vi "drawField.vi"(0 "Vision in":refnum<class "Vision.lvclass">, 1 "AutoScale":bool=TRUE, 5 "Field State Input":T12 {"Detection Frame Out"."robots_blue"."height" format="%+4.3f"; "Detection Frame Out"."robots_blue"."pixel_y" format="%+4.3f"; "Detection Frame Out"."robots_blue"."pixel_x" format="%+4.3f"; "Detection Frame Out"."robots_blue"."orientation" format="%+4.3f"; "Detection Frame Out"."robots_blue"."y" format="%+4.3f"; "Detection Frame Out"."robots_blue"."confidence" format="%4.3f"; "Detection Frame Out"."robots_blue"."x" format="%+4.3f"; "Detection Frame Out"."robots_yellow"."height" format="%+4.3f"; "Detection Frame Out"."robots_yellow"."pixel_y" format="%+4.3f"; "Detection Frame Out"."robots_yellow"."pixel_x" format="%+4.3f"; "Detection Frame Out"."robots_yellow"."orientation" format="%+4.3f"; "Detection Frame Out"."robots_yellow"."y" format="%+4.3f"; "Detection Frame Out"."robots_yellow"."confidence" format="%4.3f"; "Detection Frame Out"."robots_yellow"."x" format="%+4.3f"}, 7 "AI Parameters":T17={"GotoKick"={"Dist do cone a frente"=0.0, "attacker farback"=1300.0, "Perto"=300.0, "min dist to kick"=140.0, "kick eps"=0.15, "Time to transition"=0.3}, "Attacker"={"CC chute"=0.7, "CC passe"=0.65, "Kick Force"=85.0, "ball-robot Kick"=300.0, "ball-robot Pass"=350.0, "drible\nAttk"=FALSE}, "Defender"={"D max"=1500.0, "Vel p/ robô av"=0.2, "Kick Force"=100.0, "D atk-def"=400.0, "D farback"=300.0, "drible\ndef"=FALSE, "drible\ngoalie"=FALSE}, "Timeout"={"Field/v in x"=6.0, "Dist Robots"=300, "Dist up in y"=300}, "Pose Striker"={"dist"=650.0, "Numeric"=-4.0, "dist 2"=650.0, "drible\nstriker"=TRUE}, "Dist Stop"=700.0, "D ball out"=200, "D central gap "=125.0, "T pass"=5.0, "Force ++"=5.0, "range kick"=60.0, "Chute alto"=TRUE, "Marcador novo"=TRUE, "drible"=FALSE, "D drible"=500.0, "Versão Striker"=enum."Auto", "Defesa"=enum."ManMark", "Marcador"=enum."Marcar o mais perigoso", "Receptor passe"=enum."Auto", "Área"=enum."Circular", "Decisão\nsimples?"=FALSE} {"D drible" format="%#_13g"; "D central gap" format="%#_13g"; "Dist Stop" format="%#_13g"; "Pose Striker"."Numeric" format="%#_13g"; "Defender"."Kick Force" format="%#_13g"; "Defender"."Vel p/ robô av" format="%#_13g"; "Attacker"."ball-robot Kick" format="%#_13g"; "Attacker"."Kick Force" format="%#_13g"; "Attacker"."CC passe" format="%#_13g"; "Attacker"."CC chute" format="%#_13g"; "GotoKick"."min dist to kick" format="%#_13g"; "GotoKick"."Perto" format="%#_13g"; "GotoKick"."attacker farback" format="%#_13g"; "GotoKick"."Dist do cone a frente" format="%#_13g"}, 9 "AI State":T1={"our_robots"=[], "enemy_robots"=[], "balls"=[], "geometry"={"line_width"=0, "field_length"=0, "field_width"=0, "boundary_width"=0, "referee_width"=0, "goal_width"=0, "goal_depth"=0, "goal_wall_width"=0, "center_circle_radius"=0, "defense_radius"=0, "defense_stretch"=0, "free_kick_from_defense_dist"=0, "penalty_spot_from_field_line_dist"=0, "penalty_line_from_spot_dist"=0}, "IA Judge"={"stage"="", "command"="", "our_goalie_id"=0.0, "enemy_goalie_id"=0.0, "command enum"=enum."Halt", "Time"=enum."Azul"}, "Received Timestamp"=timestamp(0 s since 1904-01-01), "Events"={"Touch"=FALSE, "Ball out"=FALSE, "id touch"=0.0, "Ball out of \nVision"=FALSE, "Ball inside \nGoalie area"=FALSE, "Robot not responding"=FALSE, "Robots responding status"=[1.0, 1.0, 1.0, 1.0, 1.0, 1.0], "Enemy Ball \nPossession"=FALSE, "Pass State"=FALSE, "id end of pass"=0.0, "Kick"=FALSE, "Id ini Possession"=0.0, "Ball Possesion"=FALSE, "Id Possesion"=0.0, "Direct Kick"=FALSE, "2nd Strk Ativo"=FALSE}}, 11 "error in (no error)":errorcluster, 12 "Scale mm/pixel":dbl=1.0 format="%#_13g", 13 "Draw Targets?":T18, 14 "Zoom":dbl) -> (3 "AutoScale Out":bool=TRUE, 4 "Vision out":refnum<class "Vision.lvclass">, 6 "2D Picture":picture, 10 "Scale Out":dbl, 15 "error out":errorcluster)   [LabVIEW 2018, in "Vision.lvclass"]
uses:
  Vision.lvclass
  git/SSLView/DrawTargets.ctl
  git/SSLView/Intel/AI Parameters.ctl
  Old vision/Controls/SSL Field State.ctl
  Old vision/Controls/SSL Detection Frame.ctl
  Old vision/Controls/SSL Detection Robot.ctl
  <vilib>/Analysis/Matrix/Datatypes/RealMatrix.ctl
  Old vision/Controls/SSL Detection Ball.ctl
  Old vision/Controls/AI Input.ctl
  Old vision/Controls/AI Robot.ctl
  Old vision/Controls/Functions Enum.ctl
  Old vision/Controls/AttackerStates.ctl
  Old vision/Controls/PathDests.ctl
  Old vision/Controls/PathDest.ctl
  Old vision/Controls/AI Ball.ctl
  Old vision/Controls/Field Size.ctl
  Old vision/Controls/AI Judge.ctl
  Old vision/Controls/Command Enum.ctl
  Old vision/Controls/Events.ctl
  <vilib>/Utility/miscctls.llb/LVBoundsTypeDef.ctl
  <vilib>/Analysis/Matrix/NI_Matrix.lvlib
panel:
  in  "Side":enum16{"Esquerdo", "Direito"}(ring) caption="Enum"
  in  "Defense stretch":i32=500
  in  "Defense width":i32=1000
  in  "Draw Number":bool=TRUE
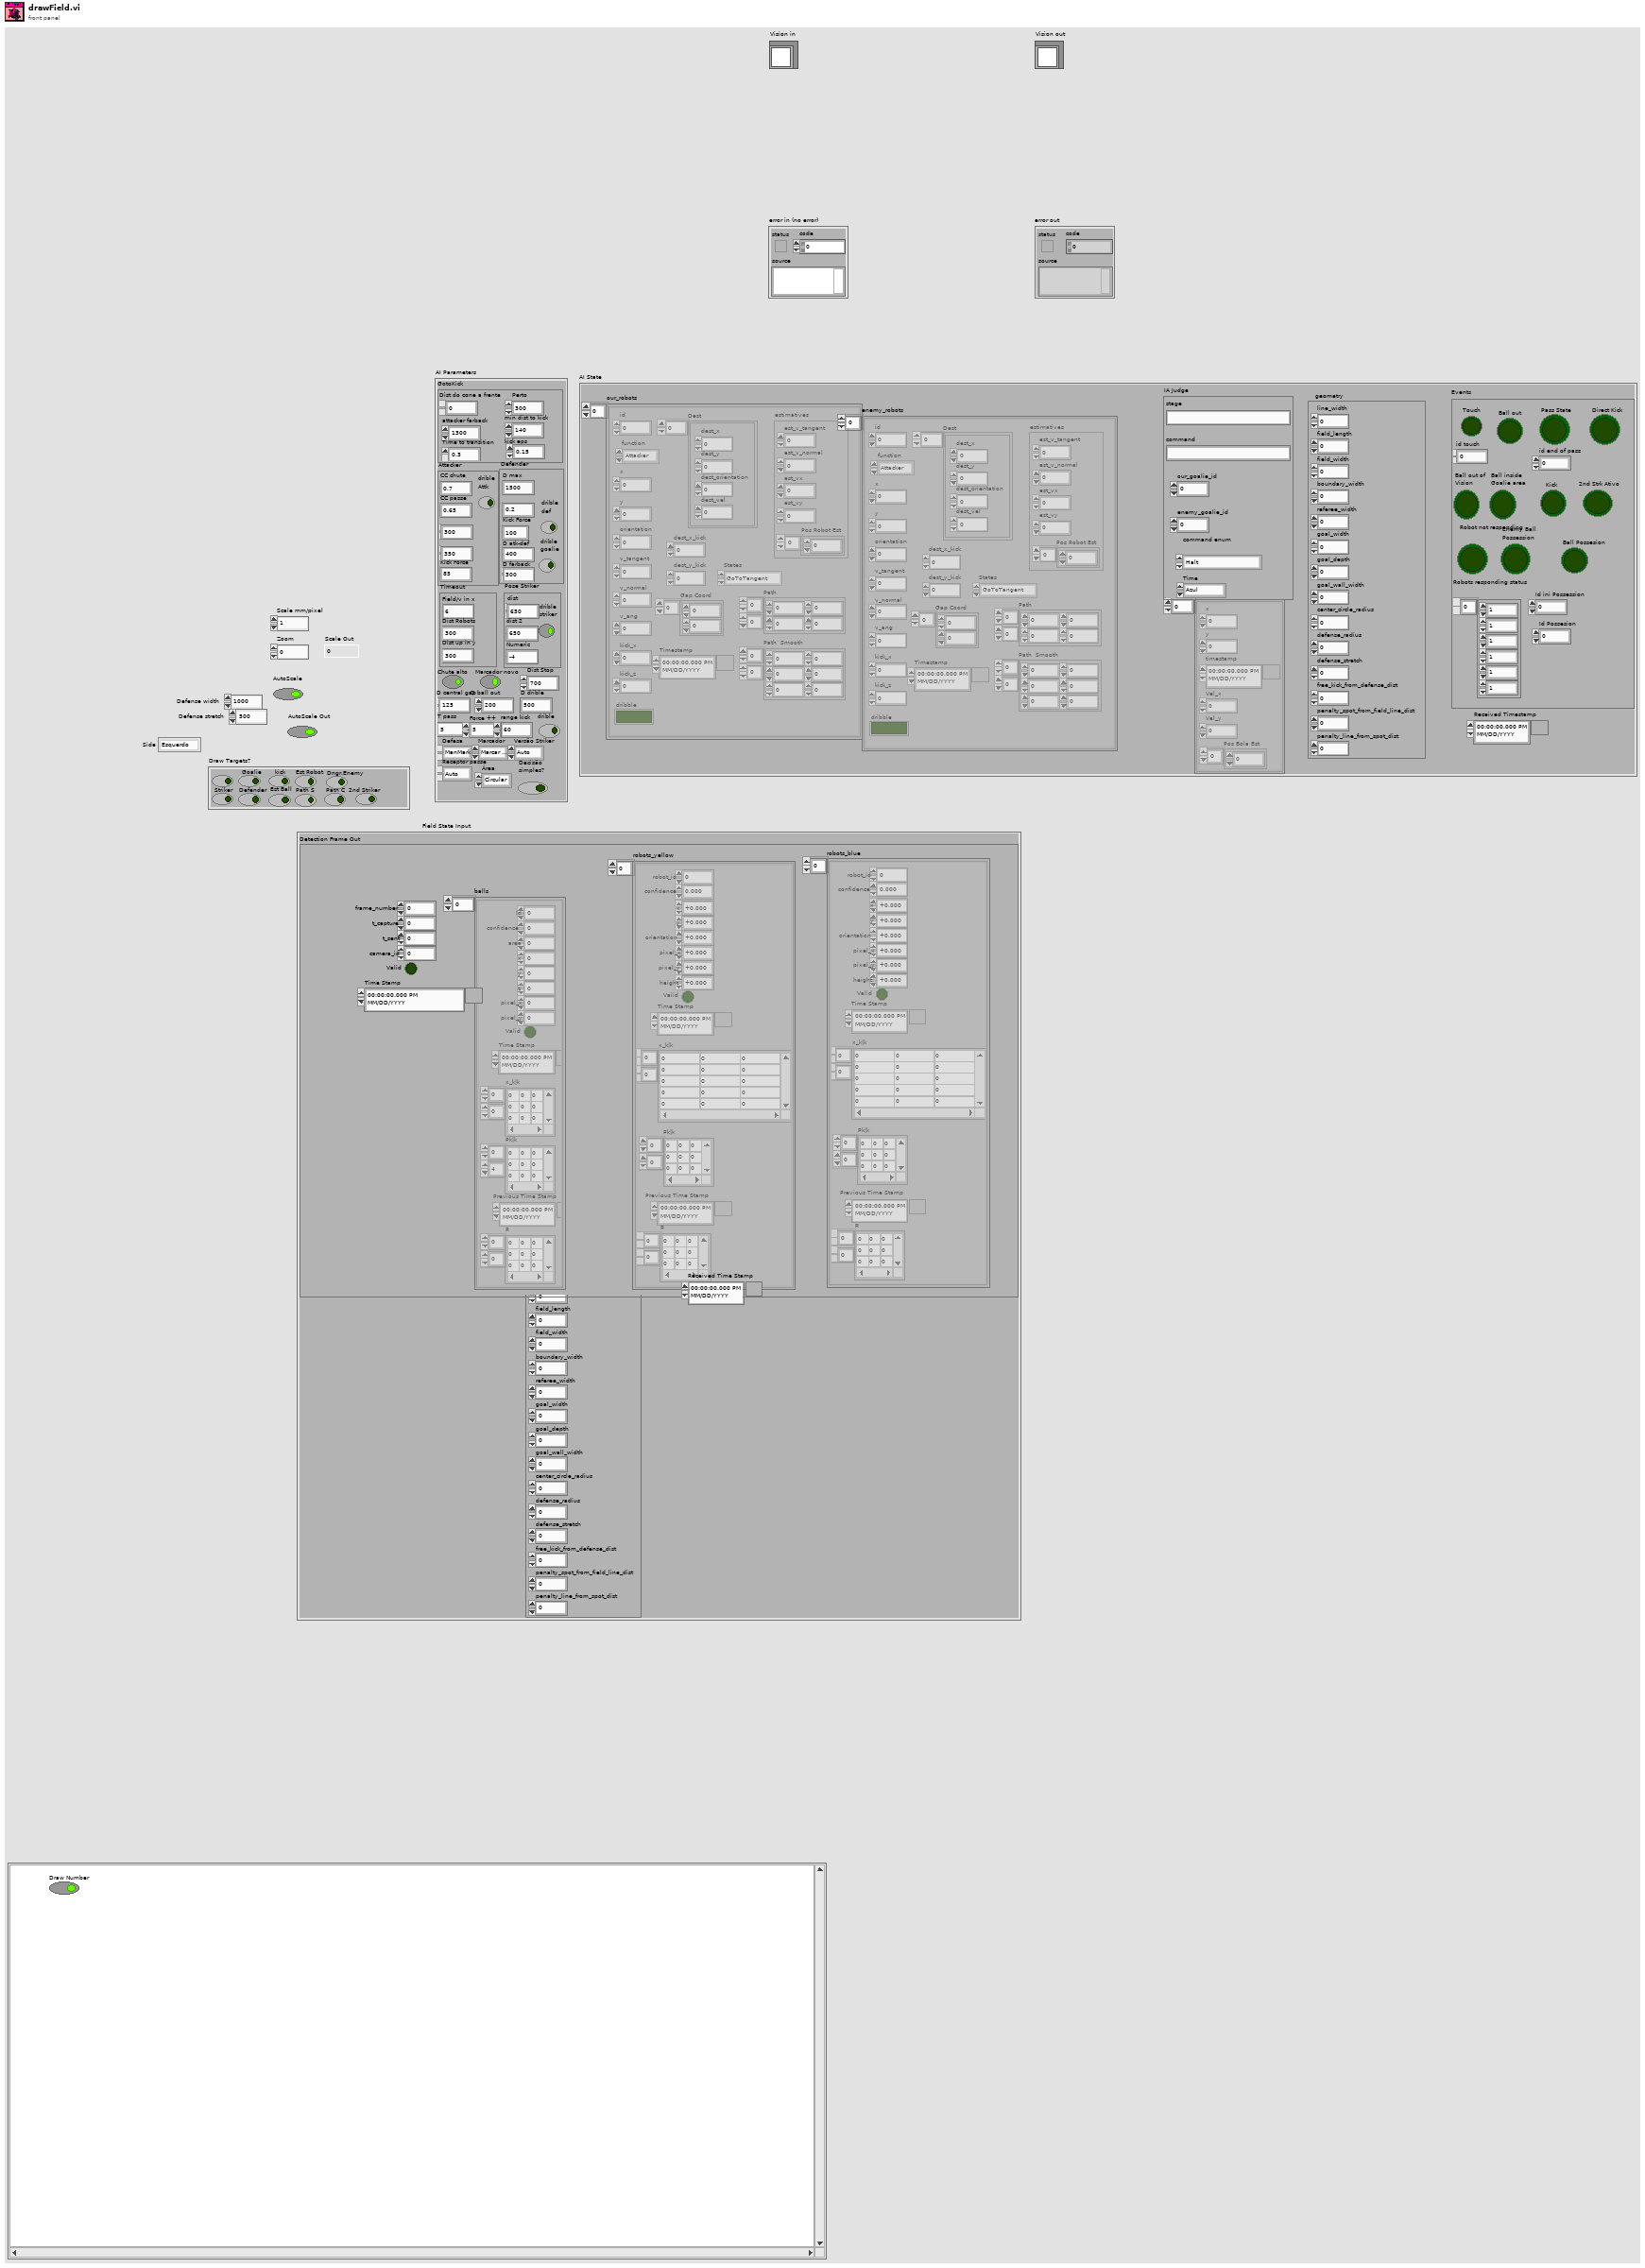
[diagram p1: front panel]
types:
  T1 = typedef "AI Input.ctl" = cluster{"our_robots":T2[], "enemy_robots":T2[], "balls":T7[], "geometry":T8, "IA Judge":T9, "Received Timestamp":timestamp, "Events":T11}
  T2 = typedef "AI Robot.ctl" = cluster{"id":u32, "function":T3, "x":dbl, "y":dbl, "orientation":dbl, "v_tangent":dbl, "v_normal":dbl, "v_ang":dbl, "kick_x":dbl, "kick_z":dbl, "dribble":bool, "Timestamp":timestamp, "estimatives":cluster{"est_v_tangent":dbl, "est_v_normal":dbl, "est_vx":dbl, "est_vy":dbl, "Pos Robot Est":dbl[]}, "dest_x_kick":dbl, "dest_y_kick":dbl, "Gap Coord":dbl[], "States":T4, "Path ":dbl[][], "Path  Smooth":dbl[][], "Dest":T5}
  T3 = typedef "Functions Enum.ctl" = enum16{"2nd Striker", "Attacker", "Goalie", "Defender", "Striker", "Goto 0", "Dummy", "Kicker", "ZigZag 0", "ZigZag 1", "ZigZag 2", "ZigZag 3", "ZigZag 4", "ZigZag 5", "ZigZag 6", "ZigZag 7", "ZigZag 8", ""}
  T4 = typedef "AttackerStates.ctl" = enum16{"Pass", "GoToTangent", "BallGetting", "GoToKick", ""}
  T5 = typedef "PathDests.ctl" = T6[]
  T6 = typedef "PathDest.ctl" = cluster{"dest_x":dbl, "dest_y":dbl, "dest_orientation":dbl, "dest_vel":dbl}
  T7 = typedef "AI Ball.ctl" = cluster{"x":dbl, "y":dbl, "timestamp":timestamp, "Vel_x":dbl, "Vel_y":dbl, "Pos Bola Est":dbl[]}
  T8 = typedef "Field Size.ctl" = cluster{"line_width":u32, "field_length":u32, "field_width":u32, "boundary_width":u32, "referee_width":u32, "goal_width":u32, "goal_depth":u32, "goal_wall_width":u32, "center_circle_radius":u32, "defense_radius":u32, "defense_stretch":u32, "free_kick_from_defense_dist":u32, "penalty_spot_from_field_line_dist":u32, "penalty_line_from_spot_dist":u32}
  T9 = typedef "AI Judge.ctl" = cluster{"stage":string, "command":string, "our_goalie_id":dbl, "enemy_goalie_id":dbl, "command enum":T10, "Time":enum16{"Azul", "Amarelo"}}
  T10 = typedef "Command Enum.ctl" = enum16{"Halt", "Stop", "Force Start", "PKA Normal Start", "Prepare Kickoff Ally", "PKE Normal Start", "Prepare Kickoff Enemy", "Prepare Penalty Ally", "PPA Normal Start", "Prepare Penalty Enemy", "PPE Normal Start", "Direct Free Enemy", "Direct Free Ally", "Indirect Free Enemy", "Indirect Free Ally", "Timeout Enemy", "Timeout Ally", "Goal Enemy", "Goal Ally", "Ball Placement Enemy", "Ball Placement Ally", "Normal Half Time", "Extra Time Break", "Extra Half Time", "None", "Post Game"}
  T11 = typedef "Events.ctl" = cluster{"Touch":bool, "Ball out":bool, "id touch":dbl, "Ball out of \nVision":bool, "Ball inside \nGoalie area":bool, "Robot not responding":bool, "Robots responding status":dbl[], "Enemy Ball \nPossession":bool, "Pass State":bool, "id end of pass":dbl, "Kick":bool, "Id ini Possession":dbl, "Ball Possesion":bool, "Id Possesion":dbl, "Direct Kick":bool, "2nd Strk Ativo":bool}
  T12 = typedef "SSL Field State.ctl" = cluster{"Detection Frame Out":T13, "Field Size Out":cluster{"line_width":u32, "field_length":u32, "field_width":u32, "boundary_width":u32, "referee_width":u32, "goal_width":u32, "goal_depth":u32, "goal_wall_width":u32, "center_circle_radius":u32, "defense_radius":u32, "defense_stretch":u32, "free_kick_from_defense_dist":u32, "penalty_spot_from_field_line_dist":u32, "penalty_line_from_spot_dist":u32}, "Received Time Stamp":timestamp}
  T13 = typedef "SSL Detection Frame.ctl" = cluster{"frame_number":u32, "t_capture":dbl, "t_sent":dbl, "camera_id":u32, "robots_yellow":T14[], "robots_blue":T14[], "balls":T16[], "Valid":bool, "Time Stamp":timestamp}
  T14 = typedef "SSL Detection Robot.ctl" = cluster{"x":sgl, "robot_id":u32, "confidence":sgl, "y":sgl, "orientation":sgl, "pixel_x":sgl, "pixel_y":sgl, "height":sgl, "Valid":bool, "Time Stamp":timestamp, "x_k|k":T15, "Pk|k":T15, "Previous Time Stamp":timestamp, "R":T15}
  T15 = typedef "NI_Matrix.lvlib/RealMatrix.ctl" = dbl[][]
  T16 = typedef "SSL Detection Ball.ctl" = cluster{"x":sgl, "area":u32, "confidence":sgl, "y":sgl, "z":sgl, "pixel_x":sgl, "pixel_y":sgl, "Valid":bool, "Time Stamp":timestamp, "x_k|k":T15, "Pk|k":T15, "Id":u32, "Previous Time Stamp":timestamp, "R":T15}
  T17 = typedef "AI Parameters.ctl" = cluster{"GotoKick":cluster{"Dist do cone a frente":dbl, "attacker farback":dbl, "Perto":dbl, "min dist to kick":dbl, "kick eps":dbl, "Time to transition":dbl}, "Attacker":cluster{"CC chute":dbl, "CC passe":dbl, "Kick Force":dbl, "ball-robot Kick":dbl, "ball-robot Pass":dbl, "drible\nAttk":bool}, "Defender":cluster{"D max":dbl, "Vel p/ robô av":dbl, "Kick Force":dbl, "D atk-def":dbl, "D farback":dbl, "drible\ndef":bool, "drible\ngoalie":bool}, "Timeout":cluster{"Field/v in x":dbl, "Dist Robots":u32, "Dist up in y":u32}, "Pose Striker":cluster{"dist":dbl, "Numeric":dbl, "dist 2":dbl, "drible\nstriker":bool}, "Dist Stop":dbl, "D ball out":i32, "D central gap ":dbl, "T pass":dbl, "Force ++":dbl, "range kick":dbl, "Chute alto":bool, "Marcador novo":bool, "drible":bool, "D drible":dbl, "Versão Striker":enum16{"Auto", "3", "2", "1"}, "Defesa":enum16{"ManMark", "Barreira"}, "Marcador":enum16{"Marcar Segundo mais perigoso", "Marcar o mais perigoso"}, "Receptor passe":enum16{"Auto", "2nd Striker", "Striker"}, "Área":enum16{"Quadrada", "Circular"}, "Decisão\nsimples?":bool}
  T18 = typedef "DrawTargets.ctl" = cluster{"Attacker":bool, "Striker":bool, "Goalie":bool, "Defender":bool, "kick":bool, "Est Ball":bool, "Est Robot":bool, "Path S":bool, "Path C":bool, "Dngr.Enemy":bool, "2nd Striker":bool}
  T19 = typedef "LVBoundsTypeDef.ctl" = cluster{"Width":u32, "Height":u32}
  T20 = cluster{"line_width":u32, "field_length":u32, "field_width":u32, "boundary_width":u32, "referee_width":u32, "goal_width":u32, "goal_depth":u32, "goal_wall_width":u32, "center_circle_radius":u32, "defense_radius":u32, "defense_stretch":u32, "free_kick_from_defense_dist":u32, "penalty_spot_from_field_line_dist":u32, "penalty_line_from_spot_dist":u32}
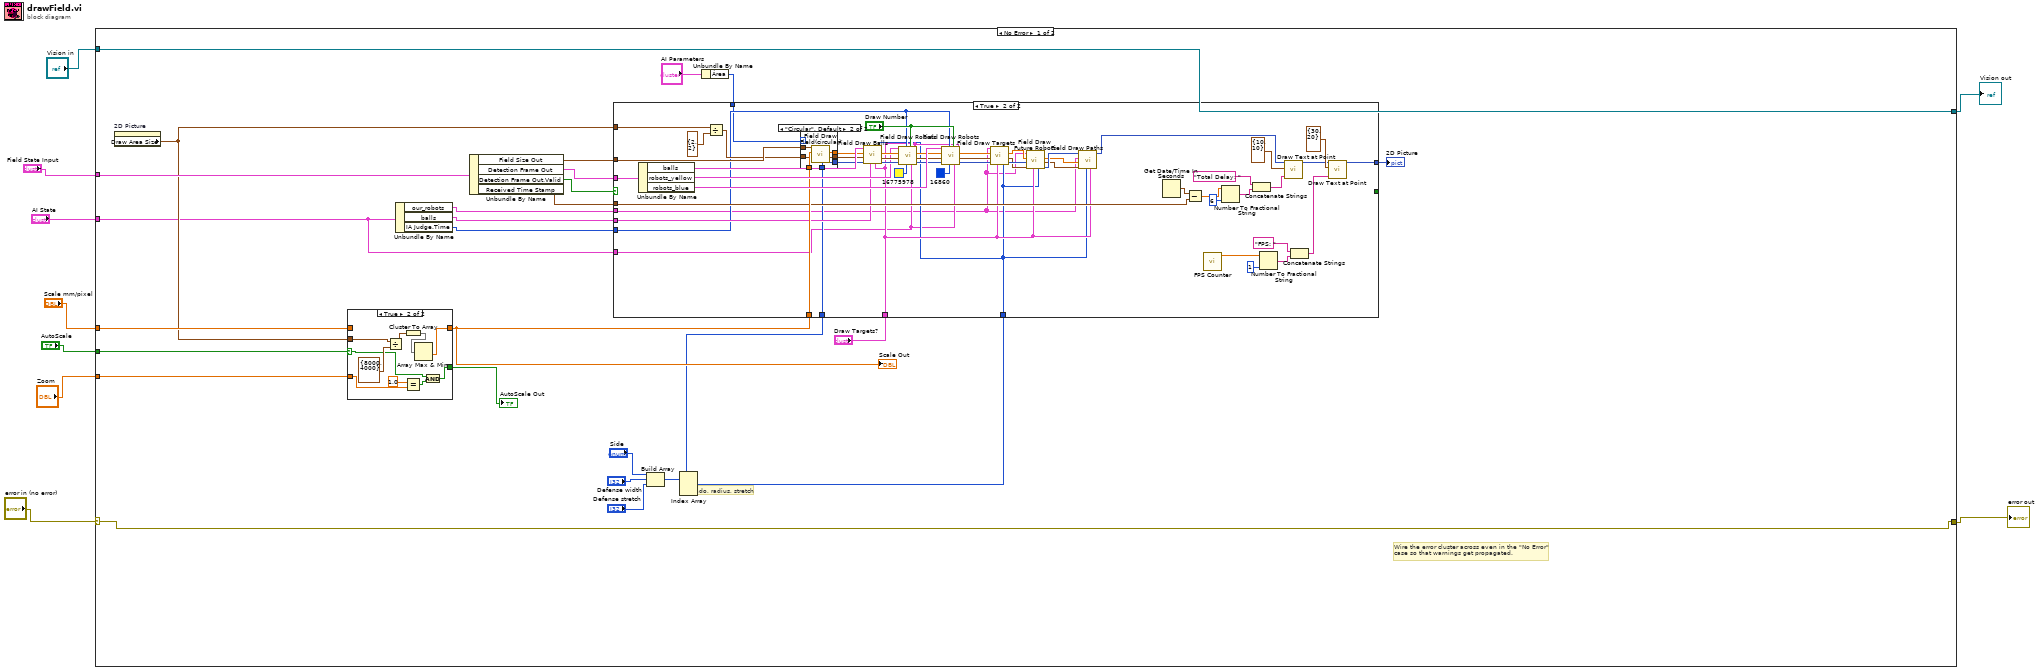
[diagram p0: block diagram]
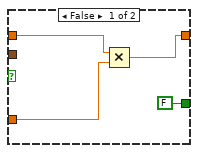
[diagram p2: hidden frame]
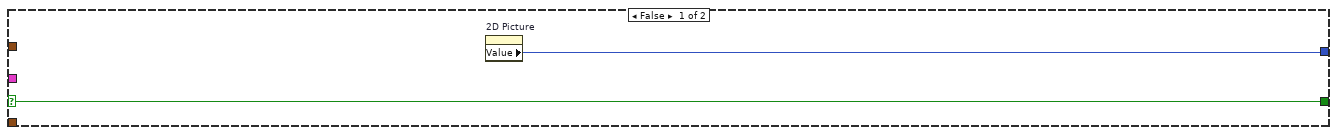
[diagram p3: hidden frame]
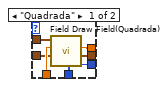
[diagram p4: hidden frame]
diagram:
  n1 = case shown="No Error" "error in (no error)" {
    selector: "error in (no error)" -> [w34 w122]
    tunnel: [w34 w122] -> w8
    tunnel: [w35 w121] -> w6
    tunnel: "Vision in" -> [w35 w121]
    tunnel: "Scale mm/pixel" -> [w24 _]
    tunnel: "AutoScale" -> [w23 _]
    tunnel: "Zoom" -> [w22 _]
    tunnel: "Field State Input" -> [w20 _]
    tunnel: "AI State" -> [w15 _]
    frame No Error {
      # "lado, radius, stretch"
      # "Wire the error cluster across even in the \"No Error\"\ncase so that warnings get propagated."
      n2 = property on="2D Picture" class="Pict"() -> ("Draw Area Size"=w16:T19)  [unwired: 2 in, 2 out]
      n3 = case shown="True" w23 {
        selector: w23 -> [_ w41]
        tunnel: w24 -> [w39 _]
        tunnel: [w38 w45] -> w14
        tunnel: w16 -> [_ w49]
        tunnel: w22 -> [w37 w44]
        tunnel: [FALSE w42] -> w21
        frame False {
          n4 = Multiply(x=w39, y=w37) -> (x*y=w38:dbl)
        }
        frame True {
          n5 = Divide(x=w49, y=T19 {"Width"=8000, "Height"=4000}) -> (x/y=w47:cluster{"Width":dbl, "Height":dbl})
          n6 = Cluster To Array(cluster=w47) -> (array=w46:dbl[])
          n7 = Equal?(x=1.0, y=w44) -> (x = y?=w40:bool)
          n8 = Array Max & Min(array=w46) -> (min value=w45:dbl)  [unwired: 3 out]
          n9 = And(x=w41, y=w40) -> (x .and. y?=w42:bool)
        }
      }
      "Scale Out" <- w14
      "AutoScale Out" <- w21
      n10 = Unbundle By Name(w15) -> ("our_robots"=w19:T2[], "balls"=w18:T7[], "IA Judge.Time"=w17:enum16{"Azul", "Amarelo"})
      n11 = Unbundle By Name(w20) -> ("Field Size Out"=w27:T20, "Detection Frame Out"=w33:T13, "Detection Frame Out.Valid"=w32:bool, "Received Time Stamp"=w31:timestamp)
      n12 = Build Array("Side", "Defense width", "Defense stretch") -> (w10:i32[])
      n13 = Index Array(array=w10) -> (element #1=w30:i32)  [unwired: 3 in, 2 out]
      n14 = Unbundle By Name("AI Parameters") -> ("Área"=w25:enum16{"Quadrada", "Circular"})
      n15 = case shown="True" w32 {
        selector: w32 -> [w51 _]
        tunnel: w16 -> [_ w105]
        tunnel: [w50 w79] -> w29
        tunnel: w33 -> [_ w93]
        tunnel: w27 -> [_ w92]
        tunnel: w14 -> [_ w91]
        tunnel: [w51 _] -> _
        tunnel: w31 -> [_ w86]
        tunnel: w19 -> [_ w54]
        tunnel: "Draw Targets?" -> [_ w58]
        tunnel: w30 -> [_ w56]
        tunnel: w18 -> [_ w69]
        tunnel: w10 -> [_ w63]
        tunnel: w17 -> [_ w62]
        tunnel: w15 -> [_ w55]
        tunnel: w25 -> [_ w53]
        frame False {
          n16 = property on="2D Picture" class="Pict"() -> ("Value"=w50:picture)  [unwired: 2 in, 2 out]
        }
        frame True {
          n17 = Unbundle By Name(w93) -> ("balls"=w104:T16[], "robots_yellow"=w100:T14[], "robots_blue"=w99:T14[])
          n18 = Divide(x=w105, y=T19 {"Width"=2, "Height"=2}) -> (x/y=w89:cluster{"Width":dbl, "Height":dbl})
          n19 = case shown="\"Circular\", Default" w53 {
            tunnel: w92 -> [w113 w120]
            tunnel: w91 -> [w112 w119]
            tunnel: [w111 w118] -> w90
            tunnel: [w107 w114] -> w52
            tunnel: w89 -> [w110 w117]
            tunnel: [w109 w116] -> w88
            tunnel: w63 -> [w108 w115]
            frame "Quadrada" {
              n20 = call "Field Draw Field(Quadrada).vi"("Lado,radius, stretch"=w108, "Offset"=w110, "Scale"=w112, "Field Size"=w113) -> ("new picture out"=w107:picture, "Offset Out"=w109:cluster{"Width":dbl, "Height":dbl}, "Scale Out"=w111:dbl)  [unwired: 5 in]
            }
            frame "Circular", Default {
              n21 = call "Field Draw Field(circular).vi"("Lado,radius, stretch"=w115, "Offset"=w117, "Scale"=w119, "Field Size"=w120) -> ("new picture out"=w114:picture, "Offset Out"=w116:cluster{"Width":dbl, "Height":dbl}, "Scale Out"=w118:dbl)  [unwired: 5 in]
            }
          }
          n22 = call "Field Draw Balls.vi"("Lado"=w56, "Draw Targets?"=w58, "balls"=w69, "Picture In"=w52, "Offset"=w88, "Scale"=w90, "Balls"=w104) -> ("Picture Out"=w103:picture, "Offset Out"=w102:cluster{"Width":dbl, "Height":dbl}, "Scale Out"=w101:dbl)  [unwired: 2 in]
          n23 = call "Field Draw Robots.vi"("Draw Targets?"=w58, "IA state"=w55, "Draw Number"="Draw Number", "color(black)"=u32 16775978, "IA Judge.Time"=w62, "Picture In"=w103, "Offset"=w102, "Scale"=w101, "Detection Robots"=w100) -> ("Picture Out"=w96:picture, "Offset Out"=w97:cluster{"Width":dbl, "Height":dbl}, "Scale Out"=w98:dbl)
          n24 = call "Field Draw Robots.vi"("Draw Targets?"=w58, "IA state"=w55, "Draw Number"="Draw Number", "color(black)"=u32 16860, "IA Judge.Time"=w62, "Picture In"=w96, "Offset"=w97, "Scale"=w98, "Detection Robots"=w99) -> ("Picture Out"=w71:picture, "Offset Out"=w70:cluster{"Width":dbl, "Height":dbl}, "Scale Out"=w68:dbl)
          n25 = call "Field Draw Targets.vi"("Lado"=w56, "Draw Targets?"=w58, "Picture In"=w71, "Offset"=w70, "Scale"=w68, "our_robots"=w54) -> ("Picture Out"=w67:picture, "Offset Out"=w66:cluster{"Width":dbl, "Height":dbl}, "Scale Out"=w65:dbl)  [unwired: 3 in]
          n26 = call "Field Draw Future Robots.vi"("Lado"=w56, "Draw Targets?"=w58, "Offset"=w66, "Picture In"=w67, "Scale"=w65, "our_robots"=w54) -> ("Picture Out"=w61:picture, "Offset Out"=w59:cluster{"Width":dbl, "Height":dbl}, "Scale Out"=w60:dbl)  [unwired: 3 in]
          n27 = call "Field Draw Paths.vi"("Draw Targets?"=w58, "Lado"=w56, "Offset"=w59, "Scale mm/pixel"=w60, "our_robots"=w54, "picture in"=w61) -> ("picture out"=w57:picture)  [unwired: 5 in]
          n28 = Get Date/Time In Seconds() -> (seconds since 1Jan1904=w85:timestamp)
          n29 = Subtract(x=w85, y=w86) -> (x-y=w84:dbl)
          n30 = call "FPS Counter.vi"() -> ("Numeric"=w75:dbl)  [unwired: 11 in]
          n31 = Number To Fractional String(number=w84, precision (6)=i16 6) -> (F-format string=w82:string)  [unwired: 2 in]
          n32 = Concatenate Strings("Total Delay: " ("text"), w82) -> (w81:string)
          n33 = Number To Fractional String(number=w75, precision (6)=i16 1) -> (F-format string=w77:string)  [unwired: 2 in]
          n34 = call <vilib>:"Draw Text at Point.vi"("text"=w81, "origin"=cluster{"x":i16, "y":i16} {"x"=10, "y"=10}, "picture"=w57) -> ("new picture"=w64:picture)  [unwired: 7 in, 1 out]
          n35 = Concatenate Strings("FPS: " ("text"), w77) -> (w73:string)
          n36 = call <vilib>:"Draw Text at Point.vi"("text"=w73, "origin"=cluster{"x":i16, "y":i16} {"x"=30, "y"=20}, "picture"=w64) -> ("new picture"=w79:picture)  [unwired: 7 in, 1 out]
        }
      }
      "2D Picture" <- w29
    }
    frame Error {
    }
  }
  "error out" <- w8
  "Vision out" <- w6
